vi "Do Run VI.vi"(8 "error in (no error)":errorcluster, 10 "Run VI Argument":T2, 11 "Data Cluster in":T1) -> (0 "error out":errorcluster, 3 "Data Cluster out":T1)   [LabVIEW 2025, in "Scripting Server.lvlib"]
uses:
  Scripting Server.lvlib
  Module Data--cluster.ctl
  Run VI (Reply Payload)--cluster.ctl
  Run VI Argument--cluster.ctl
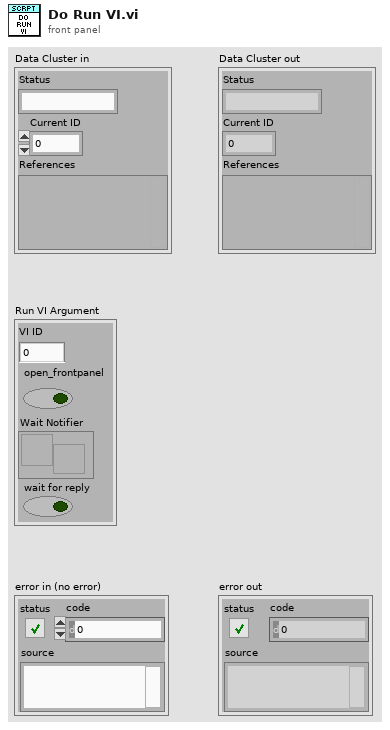
[diagram p1: front panel]
types:
  T1 = typedef "Scripting Server.lvlib/Module Data--cluster.ctl" = cluster{"Status":string, "Current ID":i32, "References":variant}
  T2 = typedef "Scripting Server.lvlib/Run VI Argument--cluster.ctl" = cluster{"VI ID":i32, "open_frontpanel":bool, "Wait Notifier":refnum<notifier>, "wait for reply":bool}
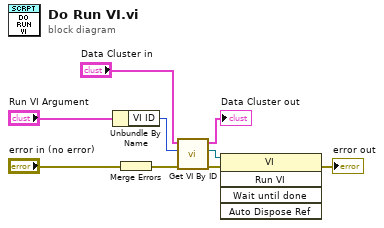
[diagram p0: block diagram]
diagram:
  n1 = Unbundle By Name("Run VI Argument") -> ("VI ID"=w3:i32)
  n2 = Merge Errors("error in (no error)") -> (w8:errorcluster)
  n3 = call "Get VI By ID.vi"("error in (no error)"=w8, "ID"=w3, "Data Cluster in"="Data Cluster in") -> ("error out"=w6:errorcluster, "VI Reference"=w1:refnum<vi>, "Data Cluster out"=→"Data Cluster out":T1)  [unwired: 6 in]
  n4 = invoke class="VI" method="Run VI"(reference=w1, error in=w6) -> (error out=→"error out":errorcluster)  [unwired: 3 in, 4 out]
